vi "List to Array.vi"(10 "List":string) -> (2 "Array":string[](array[string]))   [LabVIEW 2015, in "SLSC Switch.lvlib" / "slscsl.lvclass"]
uses:
  slscsl.lvclass
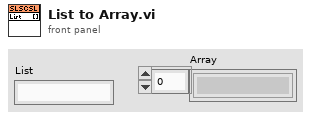
[diagram p1: front panel]
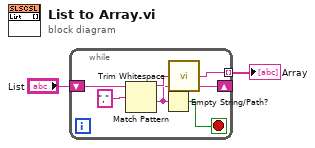
[diagram p0: block diagram]
diagram:
  n1 = while {
    tunnel: [w5] -> w1 mode=indexing
    shift-right: [w4] -> _
    shift-left: "List" -> [w7]
    stop <- w3 stop-if-true
    n2 = Match Pattern(string=w7, regular expression="," ("search string/char (-)")) -> (before substring=w6:string, after substring=w4:string)  [unwired: 1 in, 2 out]
    n3 = Empty String/Path?(string/path=w4) -> (empty?=w3:bool)
    n4 = call <vilib>:"Trim Whitespace.vi"("string"=w6) -> ("trimmed string"=w5:string)  [unwired: 1 in]
  }
  "Array" <- w1
